vi "Align.vi"(8 "error in (no error)":errorcluster, 10 "Robot":refnum<class "Robot.lvclass">, 11 "AlignSkill in":refnum<class "AlignSkill.lvclass">) -> (0 "error out":errorcluster, 2 "Robot out":refnum<class "Robot.lvclass">, 3 "AlignSkill out":refnum<class "AlignSkill.lvclass">)   [LabVIEW 2023, in "AlignSkill.lvclass"]
uses:
  AlignSkill.lvclass
  Robot_class/Robot.lvclass
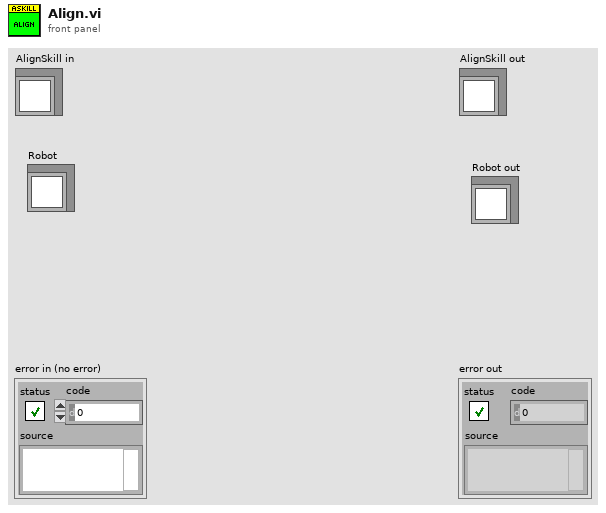
[diagram p1: front panel]
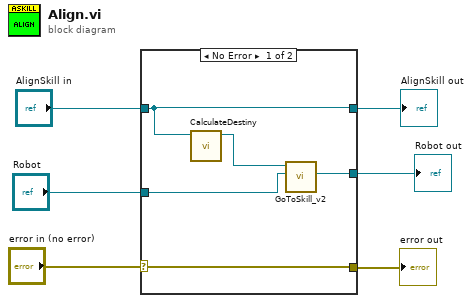
[diagram p0: block diagram]
diagram:
  n1 = case shown="No Error" "error in (no error)" {
    selector: "error in (no error)" -> [w11 w14]
    tunnel: [w11 w14] -> w5
    tunnel: [w10 w13] -> w3
    tunnel: "AlignSkill in" -> [w10 w13]
    tunnel: [w9 w12] -> w2
    tunnel: "Robot" -> [w8 w12]
    frame No Error {
      n2 = call-dynamic "CalculateDestiny.vi"("AlignSkill in"=w10) -> ("AlignSkill out"=w7:refnum<class "AlignSkill.lvclass">)  [unwired: 9 in, 1 out]
      n3 = call-dynamic "GoToSkill_v2.vi"("Robot"=w8, "object in"=w7) -> ("Robot out"=w9:refnum<class "Robot.lvclass">)  [unwired: 7 in, 2 out]
    }
    frame Error {
    }
  }
  "error out" <- w5
  "AlignSkill out" <- w3
  "Robot out" <- w2
